vi "Frequency FGV.vi"(4 "Action":enum16{"Write", "Read"}(ring)=enum."Read", 5 "error in (no error)":errorcluster, 8 "Write Value (Hz)":dbl format="%#_13g") -> (0 "error out":errorcluster, 3 "Frequency (Hz)":dbl)   [LabVIEW 2023, in "NI-568x RF Power Meter.lvlib" / "SG 2250 Path Accessor.lvclass"]
uses:
  SG 2250 Path Accessor.lvclass
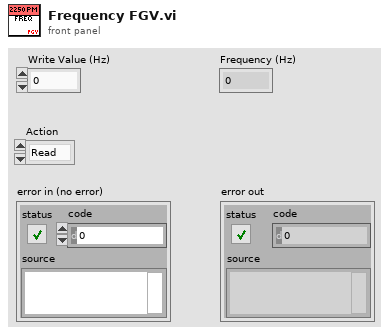
[diagram p1: front panel]
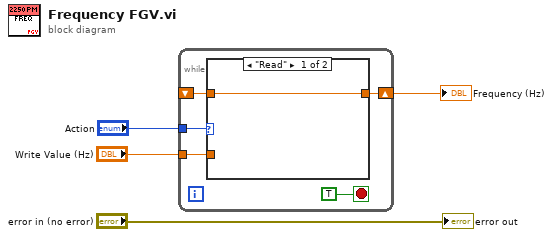
[diagram p0: block diagram]
diagram:
  n1 = while {
    tunnel: "Write Value (Hz)" -> [w7]
    shift-right: [w8] -> w3
    shift-left: _ -> [w6]
    tunnel: "Action" -> [w5]
    stop <- TRUE stop-if-true
    n2 = case shown="\"Read\"" w5 {
      tunnel: [w10 w11] -> w8
      tunnel: w7 -> [_ w11]
      tunnel: w6 -> [w10 _]
      frame "Read" {
      }
      frame "Write" {
      }
    }
  }
  "Frequency (Hz)" <- w3
  "error out" <- "error in (no error)"
